vi "SetSerializeSliceClass_StaticCommunity.vi"(8 "error in (no error)":errorcluster, 11 "BlueSerializable in":refnum<class "BlueSerializable.lvclass">) -> (0 "error out":errorcluster, 2 "Slice-To-This Class Name":string)   [LabVIEW 2020, in "BlueSerialization.lvlib" / "BlueSerializable.lvclass"]
uses:
  BlueSerializable.lvclass
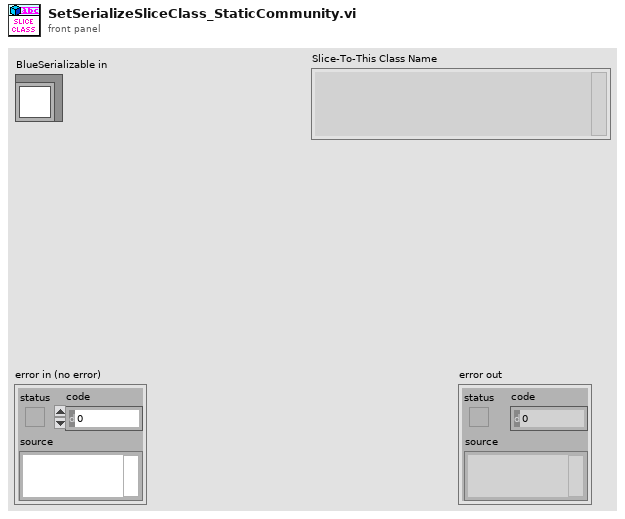
[diagram p1: front panel]
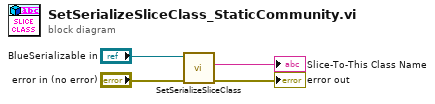
[diagram p0: block diagram]
diagram:
  n1 = call-dynamic "SetSerializeSliceClass.vi"("error in (no error)"="error in (no error)", "BlueSerializable in"="BlueSerializable in") -> ("error out"=→"error out":errorcluster, "Slice-To-This Class Name"=→"Slice-To-This Class Name":string)  [unwired: 8 in]
